vi "ConfigAI.vi"(8 "error in":errorcluster, 10 "DAQ Channels":T1=[{"DAQmx Physical"="", "Logic Name"="V", "Min Value"=-10.0, "Max Value"=10.0}], 11 "DAQ Params":T2={"Trigger Level"=1.0, "Trigger Slope"=10280, "Sample Rate"=10000.0, "N Samples"=300} {"Trigger Slope" items=["Rising"=10280, "Falling"=10171]; "Trigger Level" scale=0.0..10.0}) -> (0 "error out":errorcluster, 3 "DAQmx Task Out":refnum<k21>)   [LabVIEW 2020]
uses:
  DAQmx_Parameters.ctl
  DAQmx_Channels.ctl
  <vilib>/DAQmx/create/channels.llb/DAQmx Create Channel (AI-Voltage-Basic).vi
  <vilib>/DAQmx/configure/timing.llb/DAQmx Timing (Sample Clock).vi
  <vilib>/DAQmx/configure/trigger.llb/DAQmx Start Trigger (Analog Edge).vi
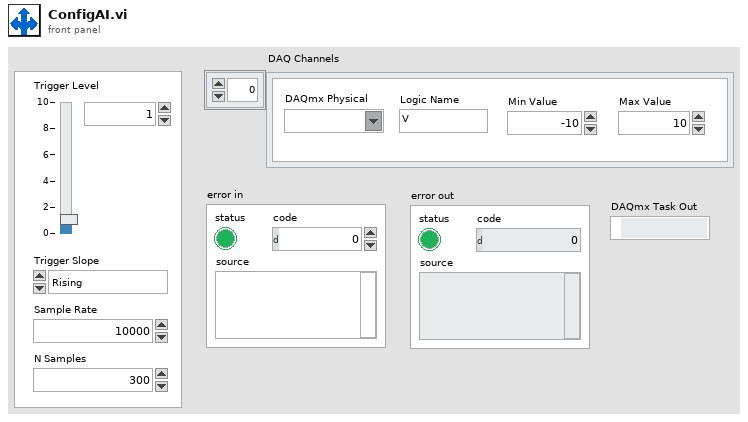
[diagram p1: front panel]
types:
  T1 = typedef "DAQmx_Channels.ctl" = cluster{"DAQmx Physical":tag, "Logic Name":string, "Min Value":dbl, "Max Value":dbl}[]
  T2 = typedef "DAQmx_Parameters.ctl" = cluster{"Trigger Level":dbl, "Trigger Slope":i32, "Sample Rate":dbl, "N Samples":i32}
  T3 = cluster{"DAQmx Physical":tag, "Logic Name":string, "Min Value":dbl, "Max Value":dbl}
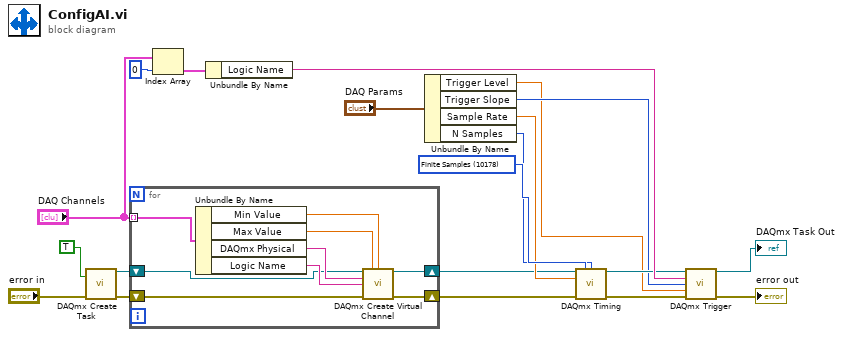
[diagram p0: block diagram]
diagram:
  w12 = 10178 items=["Finite Samples"=10178, "Continuous Samples"=10123, "Hardware Timed Single Point"=12522] ("sample mode")
  n1 = call <vilib>:"DAQmx Create Task.vi"("auto cleanup"=TRUE, "error in"="error in") -> ("task out"=w16:refnum<k21>, "error out"=w15:errorcluster)  [unwired: 12 in]
  n2 = for {
    tunnel: "DAQ Channels" -> [w29] mode=indexing
    shift-right: [w22] -> w1
    shift-left: w16 -> [w24]
    shift-right: [w21] -> w9
    shift-left: w15 -> [w23]
    n3 = Unbundle By Name(w29) -> ("Min Value"=w28:dbl, "Max Value"=w27:dbl, "DAQmx Physical"=w26:tag, "Logic Name"=w25:string)
    n4 = call-poly <vilib>:"DAQmx Create Virtual Channel.vi"("task in"=w24, "maximum value"=w27, "minimum value"=w28, "physical channels"=w26, "name to assign"=w25, "error in"=w23) -> ("task out"=w22:refnum<k21>, "error out"=w21:errorcluster)  [unwired: 8 in]
  }
  n5 = Index Array(array="DAQ Channels", index=0) -> (element=w17:T3)
  n6 = Unbundle By Name(w17) -> ("Logic Name"=w11:string)
  n7 = Unbundle By Name("DAQ Params") -> ("Trigger Level"=w3:dbl, "Trigger Slope"=w4:i32, "Sample Rate"=w6:dbl, "N Samples"=w5:i32)
  n8 = call-poly <vilib>:"DAQmx Timing.vi"("task/channels in"=w1, "sample mode"=w12, "samples per channel"=w5, "rate"=w6, "error in"=w9) -> ("task out"=w10:refnum<k21>, "error out"=w8:errorcluster)  [unwired: 9 in]
  n9 = call-poly <vilib>:"DAQmx Trigger.vi"("task/channels in"=w10, "source"=w11, "slope"=w4, "level"=w3, "error in"=w8) -> ("task out"=→"DAQmx Task Out":refnum<k21>, "error out"=→"error out":errorcluster)  [unwired: 9 in]
